vi "Teleop.vi"(10 "Match Info":T1={"Autonomous Elapsed Seconds"=0.0, "TeleOp Elapsed Seconds"=0.0, "Disabled Elapsed Seconds"=0.0, "Visited Autonomous"=FALSE, "Visited TeleOp"=FALSE, "Visited Disabled"=FALSE, "Autonomous Settings"={"Autonomous Style"=enum."Independent", "VI Refnum"=refnum}}, 11 "Call Context":T2) -> ()   [LabVIEW 2013]
doc: "This VI is called for each TeleOp packet received from the DS where the robot is not disabled. It is often used to read from the joysticks and update I/O or to update setpoints for timed control loops. It should complete and return within 20 milliseconds or it may miss DS packets."
uses:
  <vilib>/Rock Robotics/WPI/DriverStation/WPI_DriverStationDerivedRobotMode.ctl
  <vilib>/Rock Robotics/WPI/DriverStation/WPI_DriverStationMatch Info.ctl
  Begin/Robot Global Data.vi
  Begin/Global Refnums.vi
  Begin/Global Variables.vi
  <vilib>/Rock Robotics/WPI/Joystick/WPI_JoystickGetSetRefNum.vi
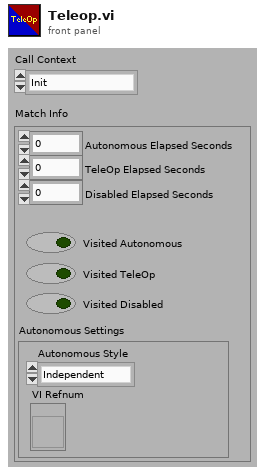
[diagram p1: front panel]
types:
  T1 = typedef "WPI_DriverStationMatch Info.ctl" = cluster{"Autonomous Elapsed Seconds":dbl, "TeleOp Elapsed Seconds":dbl, "Disabled Elapsed Seconds":dbl, "Visited Autonomous":bool, "Visited TeleOp":bool, "Visited Disabled":bool, "Autonomous Settings":cluster{"Autonomous Style":enum16{"Iterative", "Independent"}, "VI Refnum":refnum<vi>}}
  T2 = typedef "WPI_DriverStationDerivedRobotMode.ctl" = enum16{"Init", "Execute", "Stop"}
  T3 = typedef "WPI_JoystickDevRef.ctl" = cluster{"Device":T4}
  T4 = typedef "WPI_JoystickDeviceEnum.ctl" = enum16{"USB 1", "USB 2", "USB 3", "USB 4", "Kinect 1", "Kinect 2"}
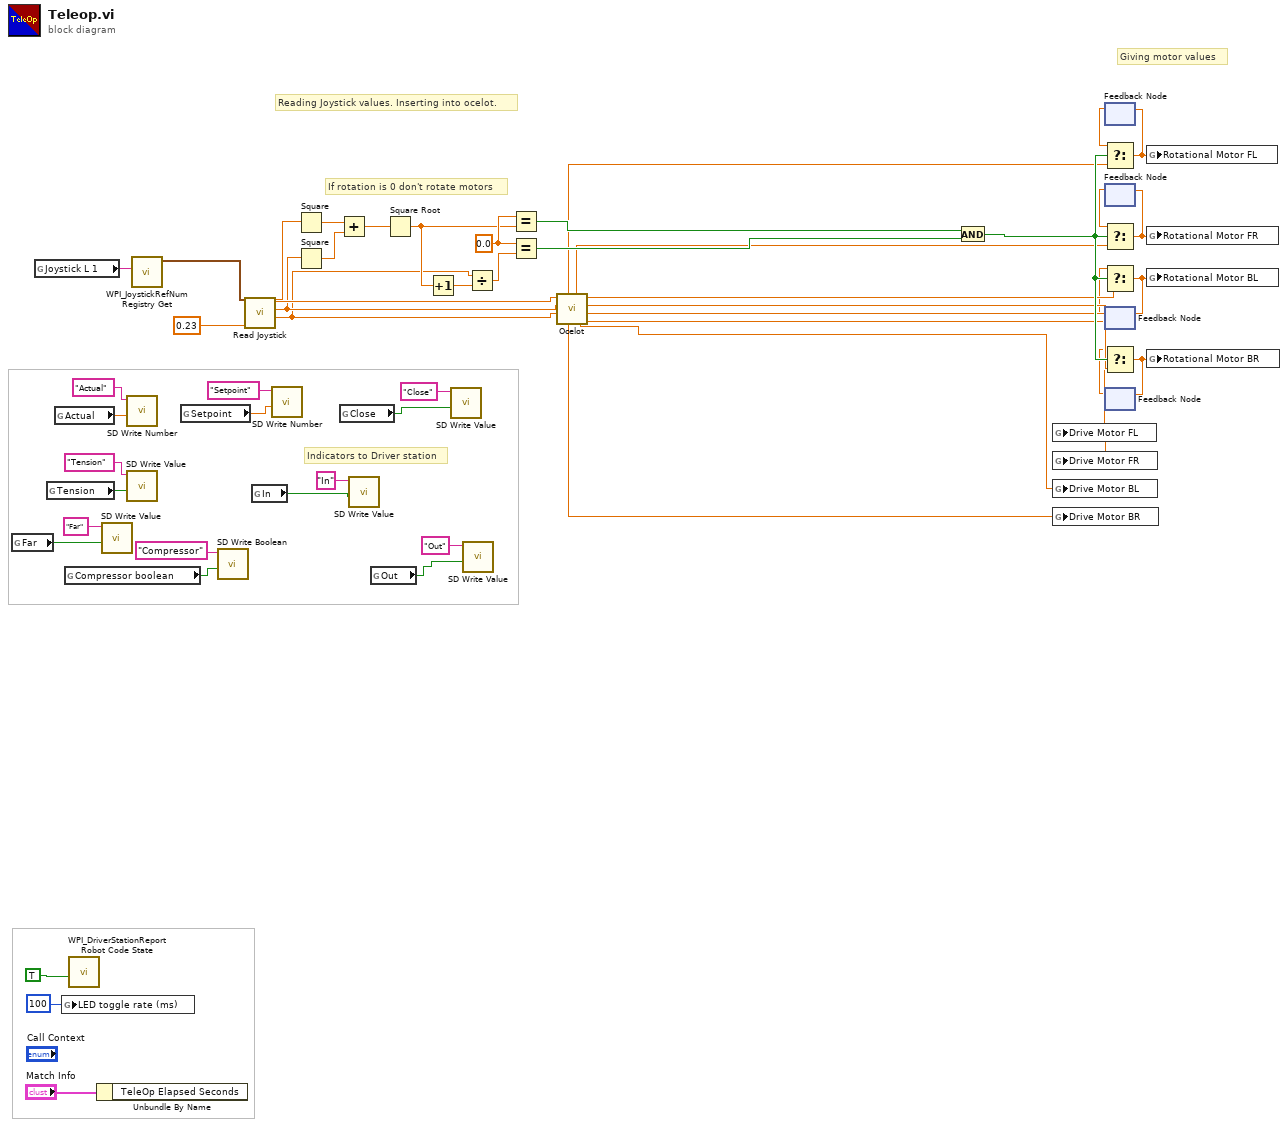
[diagram p0: block diagram]
diagram:
  w40 = 0.0 ("x")
  # "Giving motor values"
  # "If rotation is 0 don't rotate motors"
  # "Reading Joystick values. Inserting into ocelot."
  # "Indicators to Driver station"
  n1 = global read "Global Refnums.vi" "Far"() -> (w11:bool)
  n2 = global read "Global Refnums.vi" "Joystick L 1"() -> (w47:string)
  n3 = global read "Global Refnums.vi" "Tension"() -> (w15:bool)
  n4 = global read "Global Refnums.vi" "Actual"() -> (w13:dbl)
  n5 = global write "Robot Global Data.vi" "LED toggle rate (ms)"(u32 100 ("LED ms toggle rate")) -> ()
  n6 = global read "Global Refnums.vi" "Compressor boolean"() -> (w9:bool)
  n7 = call <vilib>:"WPI_DriverStationReport Robot Code State.vi"("TeleOp"=TRUE ("Autonomous")) -> ()  [unwired: 10 in, 1 out]
  n8 = Unbundle By Name("Match Info") -> ()  [unwired: 1 out]
  n9 = call-poly <vilib>:"SD Write Value.vi"("Boolean"=w11, "Name"="Far") -> ()  [unwired: 8 in, 2 out]
  n10 = call <vilib>:"SD Write Number.vi"("Numeric"=w13, "Name"="Actual") -> ()  [unwired: 8 in, 2 out]
  n11 = call-poly <vilib>:"SD Write Value.vi"("Boolean"=w15, "Name"="Tension") -> ()  [unwired: 8 in, 2 out]
  n12 = call <vilib>:"WPI_JoystickRefNum Registry Get.vi"("refnum name"=w47) -> ("JoystickDevRef"=w17:T3)  [unwired: 9 in, 1 out]
  n13 = global read "Global Refnums.vi" "Setpoint"() -> (w1:dbl)
  n14 = call <vilib>:"SD Write Boolean.vi"("Boolean"=w9, "Name"="Compressor") -> ()  [unwired: 8 in, 2 out]
  n15 = call "Read Joystick.vi"("Joystick Deadbanded Value (default of 0.1)"=0.23, "Joystick L 1 DevRef"=w17) -> ("Joystick R 2 X Axis"=w34:dbl, "Joystick L 1 Y Axis"=w35:dbl, "Joystick L 1 X Axis"=w36:dbl)  [unwired: 7 in]
  n16 = global read "Global Refnums.vi" "In"() -> (w7:bool)
  n17 = call <vilib>:"SD Write Number.vi"("Numeric"=w1, "Name"="Setpoint") -> ()  [unwired: 8 in, 2 out]
  n18 = Square(x=w36) -> (x^2=w45:dbl)
  n19 = Square(x=w35) -> (x^2=w46:dbl)
  n20 = Add(x=w45, y=w46) -> (x+y=w44:dbl)
  n21 = global read "Global Refnums.vi" "Close"() -> (w3:bool)
  n22 = call-poly <vilib>:"SD Write Value.vi"("Boolean"=w7, "Name"="In") -> ()  [unwired: 8 in, 2 out]
  n23 = global read "Global Refnums.vi" "Out"() -> (w5:bool)
  n24 = Square Root(x=w44) -> (sqrt(x)=w38:dbl)
  n25 = Increment(x=w38) -> (x+1=w39:dbl)
  n26 = call-poly <vilib>:"SD Write Value.vi"("Boolean"=w3, "Name"="Close") -> ()  [unwired: 8 in, 2 out]
  n27 = call-poly <vilib>:"SD Write Value.vi"("Boolean"=w5, "Name"="Out") -> ()  [unwired: 8 in, 2 out]
  n28 = Divide(x=w34, y=w39) -> (x/y=w37:dbl)
  n29 = Equal?(x=w40, y=w38) -> (x = y?=w42:bool)
  n30 = Equal?(x=w40, y=w37) -> (x = y?=w41:bool)
  n31 = call "Ocelot.vi"("RCW (X2)"=w34, "FWD (Y)"=w35, "STR (X)"=w36) -> ("FRD"=w28:dbl, "FLD"=w29:dbl, "BRS"=w30:dbl, "BLS"=w31:dbl, "BLD"=w27:dbl, "FRS"=w32:dbl, "BRD"=w26:dbl, "FLS"=w33:dbl)  [unwired: 1 in]
  n32 = And(x=w42, y=w41) -> (x .and. y?=w43:bool)
  n33 = global write "Global Variables.vi" "Drive Motor FL"(w29) -> ()
  n34 = global write "Global Variables.vi" "Drive Motor FR"(w28) -> ()
  n35 = global write "Global Variables.vi" "Drive Motor BL"(w27) -> ()
  n36 = global write "Global Variables.vi" "Drive Motor BR"(w26) -> ()
  n37 = feedback #1() -> (w25:dbl)  [unwired: 1 in]
  n38 = Select(t=w25, s=w43, f=w33) -> (s? t:f=w19:dbl)
  n39 = feedback-in #1(w19) -> ()
  n40 = feedback #2() -> (w24:dbl)  [unwired: 1 in]
  n41 = Select(t=w24, s=w43, f=w32) -> (s? t:f=w21:dbl)
  n42 = feedback-in #2(w21) -> ()
  n43 = feedback #3() -> (w23:dbl)  [unwired: 1 in]
  n44 = Select(t=w23, s=w43, f=w31) -> (s? t:f=w20:dbl)
  n45 = feedback-in #3(w20) -> ()
  n46 = feedback #4() -> (w22:dbl)  [unwired: 1 in]
  n47 = Select(t=w22, s=w43, f=w30) -> (s? t:f=w18:dbl)
  n48 = feedback-in #4(w18) -> ()
  n49 = global write "Global Variables.vi" "Rotational Motor FL"(w19) -> ()
  n50 = global write "Global Variables.vi" "Rotational Motor FR"(w21) -> ()
  n51 = global write "Global Variables.vi" "Rotational Motor BL"(w20) -> ()
  n52 = global write "Global Variables.vi" "Rotational Motor BR"(w18) -> ()
